vi "Read Image.vi"(8 "error in (no error)":errorcluster, 11 "Storage in":refnum<class "Storage.lvclass">) -> (0 "error out":errorcluster, 2 "Image":T1, 3 "Storage out":refnum<class "Storage.lvclass">)   [LabVIEW 2014, in "Storage.lvlib" / "Storage.lvclass"]
uses:
  Storage.lvclass
  <vilib>/vision/Image Controls.llb/IMAQ Image.ctl
  Storage.lvclass/Storage.ctl
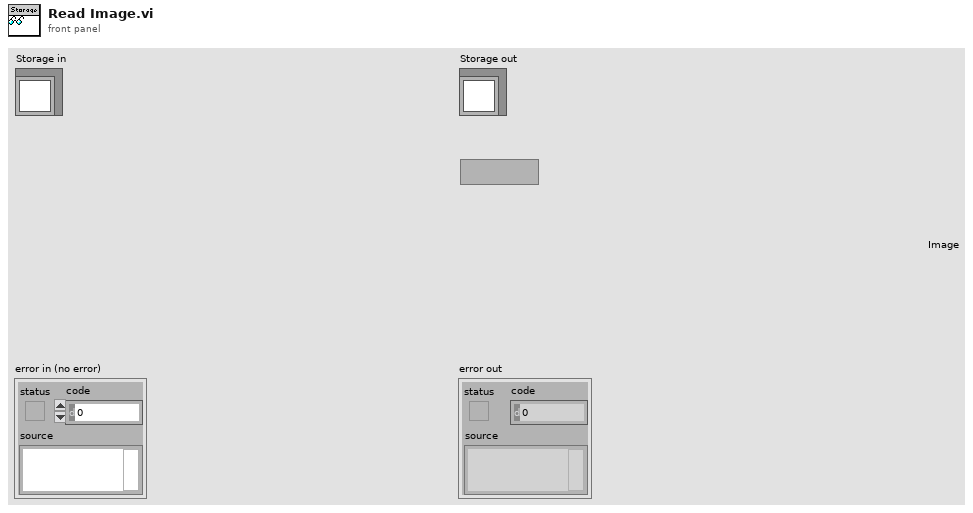
[diagram p1: front panel]
types:
  T1 = typedef "IMAQ Image.ctl" = refnum<image>
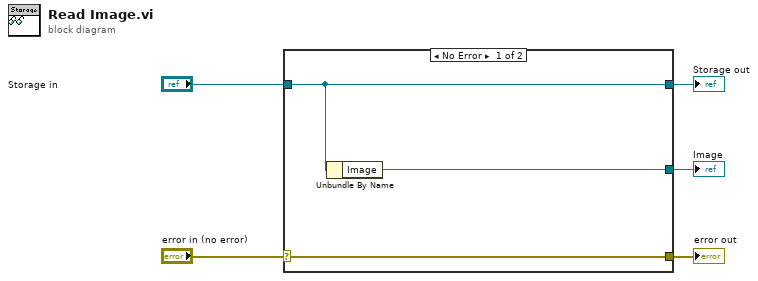
[diagram p0: block diagram]
diagram:
  n1 = case shown="No Error" "error in (no error)" {
    selector: "error in (no error)" -> [w8 w9]
    tunnel: [w8 w9] -> w4
    tunnel: [w7 w10] -> w2
    tunnel: "Storage in" -> [w7 w10]
    tunnel: [w6 _] -> w1
    frame No Error {
      n2 = Unbundle By Name(w7) -> ("Image"=w6:T1)
    }
    frame Error {
    }
  }
  "error out" <- w4
  "Storage out" <- w2
  "Image" <- w1
